vi "instrumentProperties_status.vi"(0 "reference":refnum<class "OSA.lvclass">, 5 "error in (no error)":errorcluster, 7 "poll update":bool) -> (9 "update":bool, 14 "duplicate reference":refnum<class "OSA.lvclass">, 16 "status code":u32, 17 "status":string, 18 "status struct":T1, 19 "error out":errorcluster)   [LabVIEW 2010, in "OSA.lvclass"]
doc: "Nr of samples per period depends on sensitivity mode."
uses:
  OSA.lvclass
  typeDef/status.ctl
  FTSLib.dll
  OSA20X_misc.lvlib
panel:
  out "x*2^n":u32 format="%x"
  in  "poll timeout (30s)":i32=30
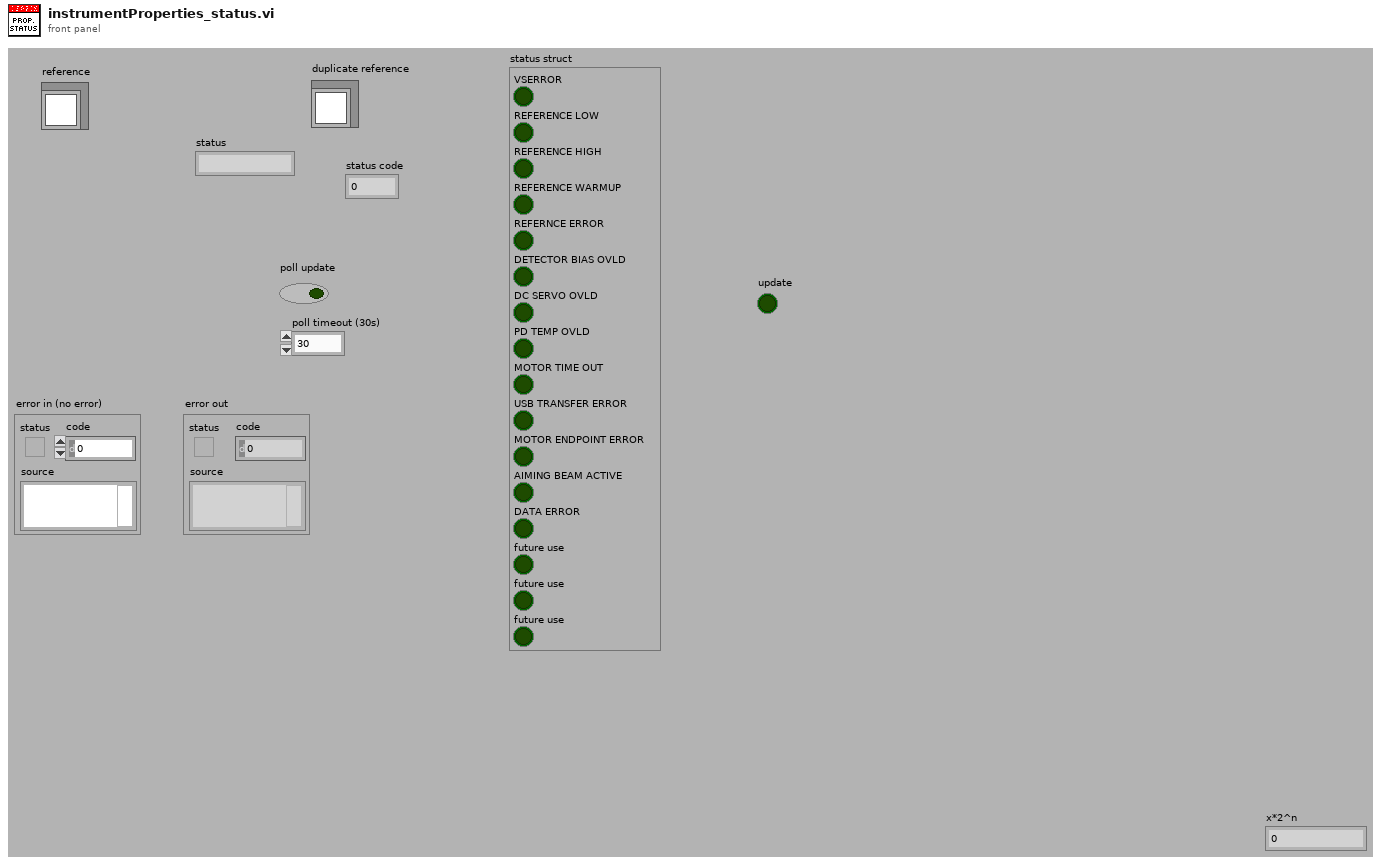
[diagram p1: front panel]
types:
  T1 = cluster{"VSERROR":bool, "REFERENCE LOW ":bool, "REFERENCE HIGH ":bool, "REFERENCE WARMUP ":bool, "REFERNCE ERROR ":bool, "DETECTOR BIAS OVLD":bool, "DC SERVO OVLD":bool, "PD TEMP OVLD":bool, "MOTOR TIME OUT":bool, "USB TRANSFER ERROR":bool, "MOTOR ENDPOINT ERROR":bool, "AIMING BEAM ACTIVE":bool, "DATA ERROR":bool, "future use":bool, "future use":bool, "future use":bool}
  T2 = typedef "OSA.lvclass/status.ctl" = cluster{"code":u32, "string":string}
  T3 = cluster{"Boolean array[0]":bool, "Boolean array[1]":bool, "Boolean array[2]":bool, "Boolean array[3]":bool, "Boolean array[4]":bool, "Boolean array[5]":bool, "Boolean array[6]":bool, "Boolean array[7]":bool, "Boolean array[8]":bool, "Boolean array[9]":bool, "Boolean array[10]":bool, "Boolean array[11]":bool, "Boolean array[12]":bool, "Boolean array[13]":bool, "Boolean array[14]":bool, "Boolean array[15]":bool}
  T4 = typedef "OSA.lvclass/ObjectAttributes.ctl" = cluster{"Stop":bool, "dataType":T5, "spectrometerIdx":u16, "buffer size interferogram":i32, "interferogram":cluster{"new":bool, "plot_x_ min":sgl, "plot_x_max":sgl, "plot_y_min":sgl, "plot_y_max":sgl, "Graph Intrfrgrm":T6, "timeStamp":u32, "signal (%)":dbl, "traces":cluster{"idx":u32, "broadBand":bool, "monoChromatic":bool, "peakToPeakSignal":dbl, "peakToPeakPos":dbl}[], "traces idx last":i32}, "spectrum":cluster{"new":bool, "plot_x_min":sgl, "plot_x_max":sgl, "plot_unit_x":T7, "plot_unit_y":T8, "plot_y_min":sgl, "plot_y_max":sgl, "Graph Spectrum":T6, "timeStamp":u32, "X_VAL_OPTIONS":enum16{"MIN_MAX", "ARRAY"}, "traces":cluster{"idx":u32}[], "traces idx last":i32}, "Thorlabs_OSA_64.lvclass:queue_action.ctlqueue ref":refnum<queue>, "action":T9, "plot zoom step":dbl, "buffer semaphore":T10, "acq stopped":bool, "dataType active":T5, "temperature (degr C)":sgl, "pressure (hPa)":sgl, "rel humidity (%)":sgl, "settings":cluster{"resolution":u16, "sensitivity":u16, "Average":bool, "average nr":u32, "apodisation":T11, "acq delay (ms)":u32, "airMesure":T12, "wmtr on":bool, "intfgrm_smooth_width":u16, "intfgrm_smooth_nrOfPasses":u16, "intfgrm_smooth":T13, "phaseCorrection":T14, "zeroFill":u8, "spectr_smooth":T13, "spectr_smooth_width":u16, "spectr_smooth_nrOfPasses":u16, "resolution (/cm)":sgl, "REF wavelength, (nm)":dbl, "gain_idx":u16, "gainAuto":bool, "gain_relative":dbl, "PD sensitivity mode":T15, "PD senseMode implemented":bool, "SensorTemperature implemented":bool, "SensorPressure implemented":bool, "SensorHumidity implemented":bool, "attenuationAuto":bool, "attenuationOnOff":bool, "attenuationAvailable":bool, "offsetAvailable":bool, "offset":i32, "offset max":u16}, "peaks position":sgl[], "peaks width":sgl[], "peaks height":sgl[], "peaks max nr":u32, "peaks latest nr":i32, "peaks new":bool, "power":dbl, "power new":bool, "path":string, "wavelength (WNr)":dbl, "wavelength new":bool, "buffer size spectrum":i32, "status":string, "VI reference":refnum<vi>, "funcPointer":u64, "libraryPointer":u64, "singleAcquisition":bool, "coherenceLength (cm)":dbl, "coherenceLength new":bool, "spectrometer model":string, "spectrometer serial nr":string, "peaks thld left":sgl[], "peaks thld right":sgl[], "coherenceLength error (cm)":dbl, "ADC bits":u16, "peaks position centroid":sgl[], "peaks height centroid":sgl[], "OSA series":T16, "channel index spectrum":u16, "spectrometer rangeLow, (/cm)":dbl, "spectrometer rangeHigh, (/cm)":dbl, "channel index interferogram":u16}
  T5 = typedef "OSA.lvclass/acq_dataType.ctl" = enum16{"none", "interferogram", "spectrum"}
  T6 = typedef "OSA.lvclass/graph_intensity.ctl" = refnum<vi>
  T7 = typedef "OSA.lvclass/spectrum_x_unit.ctl" = enum16{"wavenr/cm", "THz", "eV", "nm_air", "nm_vac"}
  T8 = typedef "OSA.lvclass/y_unit.ctl" = enum16{"ADC counts", "dBm pwr absolute", "dBm pwr density", "mW pwr absolute", "mW pwr density"}
  T9 = typedef "OSA.lvclass/queue_action.ctl" = enum16{"none", "stop", "GUI_plotInterferogram", "GUI_plotSpectrum", "GUI_plotInterferogramRescale", "GUI_plotSpectrumRescale", "GUI_plotInterferogramReset", "GUI_plotSpectrumReset", "GUI_plotInterferogramAutoScaleY", "GUI_plotSpectrumAutoScaleY", "GUI_plotInterferogramZoomOut", "GUI_plotSpectrumZoomOut", "GUI_plotInterferogramPane", "GUI_plotSpectrumPane", "GUI_plotInterferogramZoomMouse", "GUI_plotSpectrumZoomMouse", "GUI_spectrumChannelType", "GUI_channel", "ENVIRONMENT temperature", "ENVIRONMENT pressure", "MODE_resolution set", "MODE_resolution get", "MODE_sensitivity set", "MODE_sensitivity get", "MODE_PDTemperature set", "MODE_PDTemperature get", "REBOOT/RESET firmware", "ACQASYNC_acquireSingleSpectrum", "ACQASYNC_continuous start", "ACQASYNC_continuous stop\n", "ACQASYNC_get last interferogram", "ACQASYNC_get last spectrum", "ACQASYNC_get last waveNr", "ACQOPT_interferogram smoothing set", "ACQOPT_interferogram smoothing get", "ACQOPT_spectrum smoothing set", "ACQOPT_spectrum smoothing get", "ACQOPT_apodisation type set", "ACQOPT_apodisation type get", "ACQOPT_phase correction type set", "ACQOPT_phase correction type get", "ACQOPT_acqIntervall_set", "ACQOPT_acqIntervall_get", "ACQOPT_average spectrum set", "ACQOPT_average spectrum get", "ACQOPT_rolling average set", "ACQOPT_rolling average get", "ACQOPT_zero fill factor set", "ACQOPT_zero fill factor get", "ACQOPT_cycle counting set", "ACQOPT_cycle counting get", "ACQOPT_air measure option set", "ACQOPT_air measure option get", "ACQOPT_gainLevel auto get", "ACQOPT_gainLevel auto set", "ACQOPT_gainLevel get", "ACQOPT_gainLevel set", "ACQOPT_getAll", "INSTRUMENT_PROPERTY_range_WaveNr_min", "INSTRUMENT_PROPERTY_range_WaveNr_max", "INSTRUMENT_PROPERTY_reference_wavelength_cm^-1", "INSTRUMENT_PROPERTY_samplesPerRefPeriod", "INSTRUMENT_PROPERTY_resolution_waveNrPercm", "INSTRUMENT_PROPERTY_availableGainLevels", "INSTRUMENT_PROPERTY_status", "CONVERT", "ANALYSE_POWER", "ANALYSE_PEAKS", "ANALYSE_WAVELENGTH", "ANALYSE_SPECTRUM", "ANALYSE_INTERFEROGRAM", "ANALYSE_COHERENCE_LENGTH", "MATH", "MATH_power", "MATH_peaks", "FILE", "miscellaneous"}
  T10 = typedef "Semaphore RefNum" = refnum<k1>
  T11 = typedef "OSA.lvclass/apodisation.ctl" = enum16{"NONE", "NORTON_BEER_WEAK", "NORTON_BEER_MEDIUM", "NORTON_BEER_STRONG", "TRIANGULAR", "COSINE", "HANN", "HAMMING", "BLACKMANHARRIS3", "BLACKMANHARRIS4", "GAUSSIAN"}
  T12 = typedef "OSA.lvclass/airMeasure.ctl" = enum16{"TEMPERATURE", "PRESSURE"}
  T13 = typedef "OSA20X_misc.lvlib/interferogram_smoothing.ctl" = enum16{"NONE", "BINOMIAL", "SAVITSKY_GOLAY", "FOURIER", "MOVING_AVERAGE", "GAUSSIAN"}
  T14 = typedef "OSA.lvclass/phaseCorrection.ctl" = enum16{"NONE", "MERTZ", "FORMAN", "MERTZ_FILE", "FORMAN_FILE", "FUTURE COMP."}
  T15 = typedef "OSA20X_misc.lvlib/PDTemperatureMode.ctl" = enum16{"cool: better sensitivity/noise floor", "warm: extended wl range"}
  T16 = typedef "OSA.lvclass/OSA_series.ctl" = enum16{"OSA200", "OSA300", "UNKNOWN"}
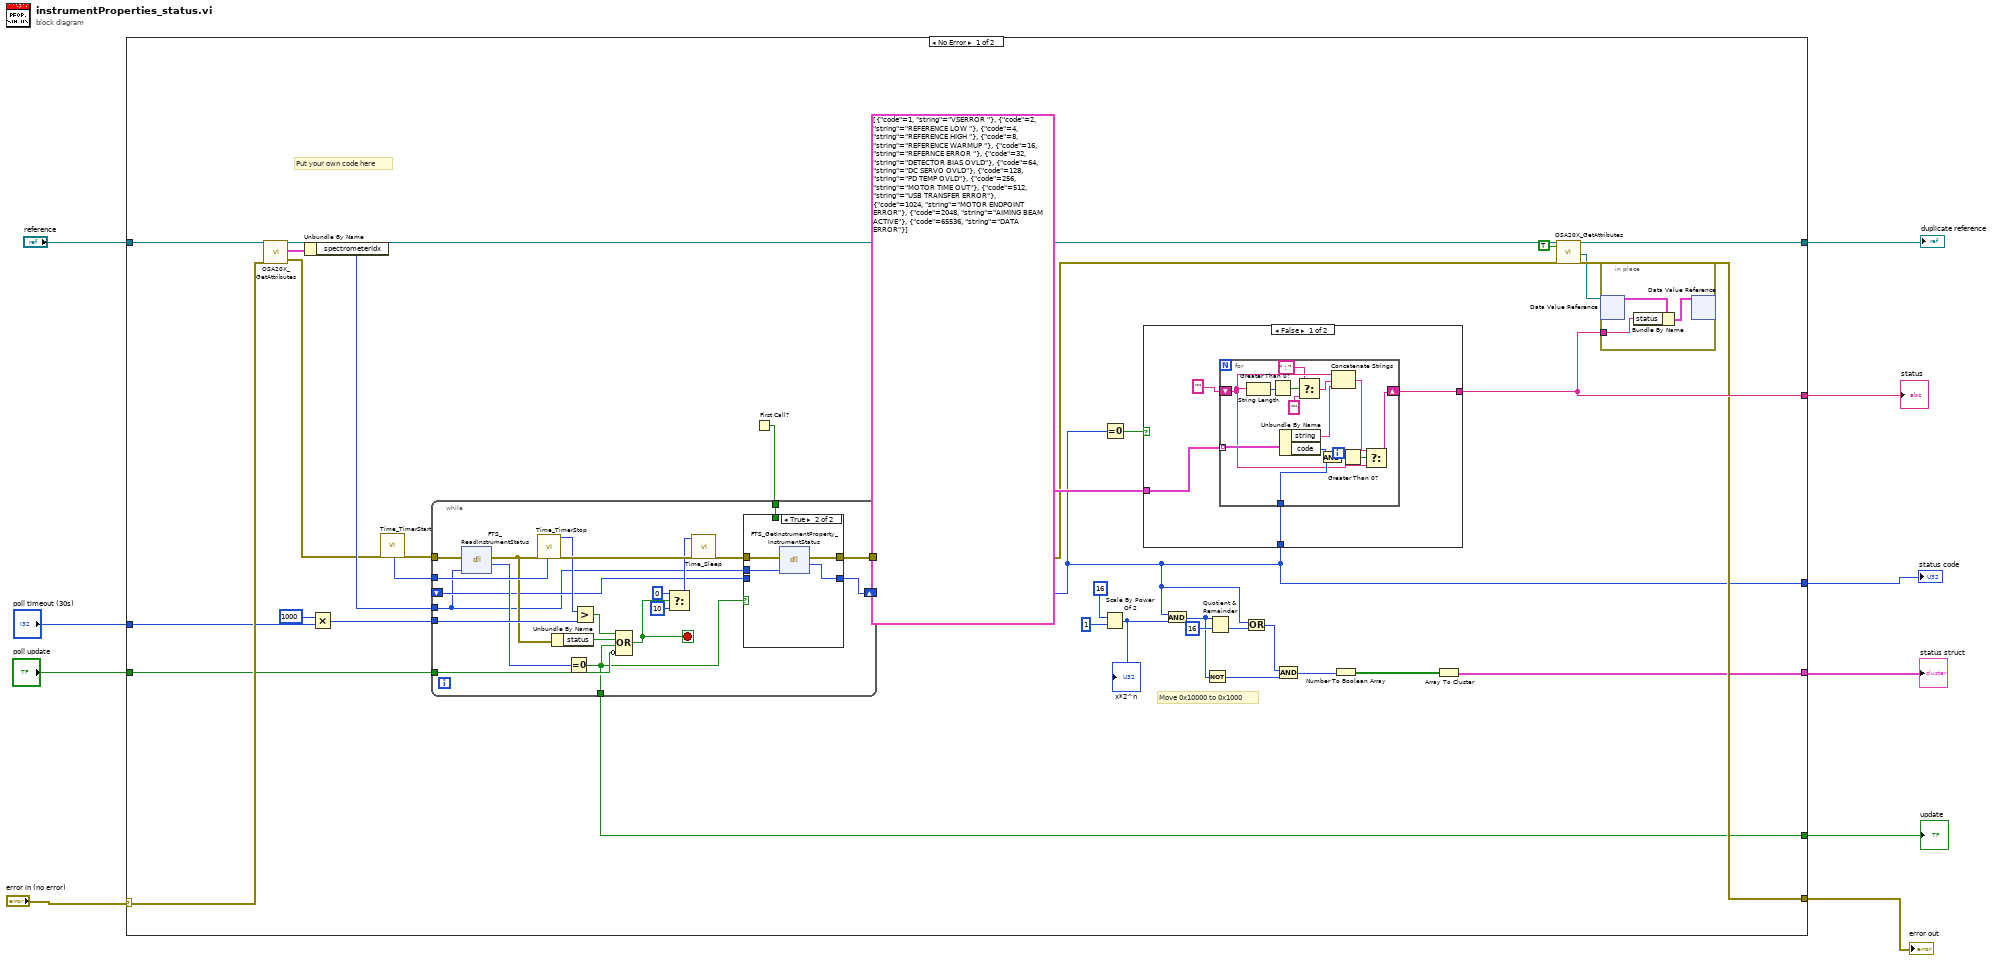
[diagram p0: block diagram]
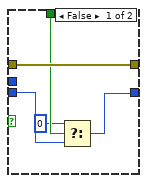
[diagram p2: hidden frame]
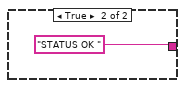
[diagram p3: hidden frame]
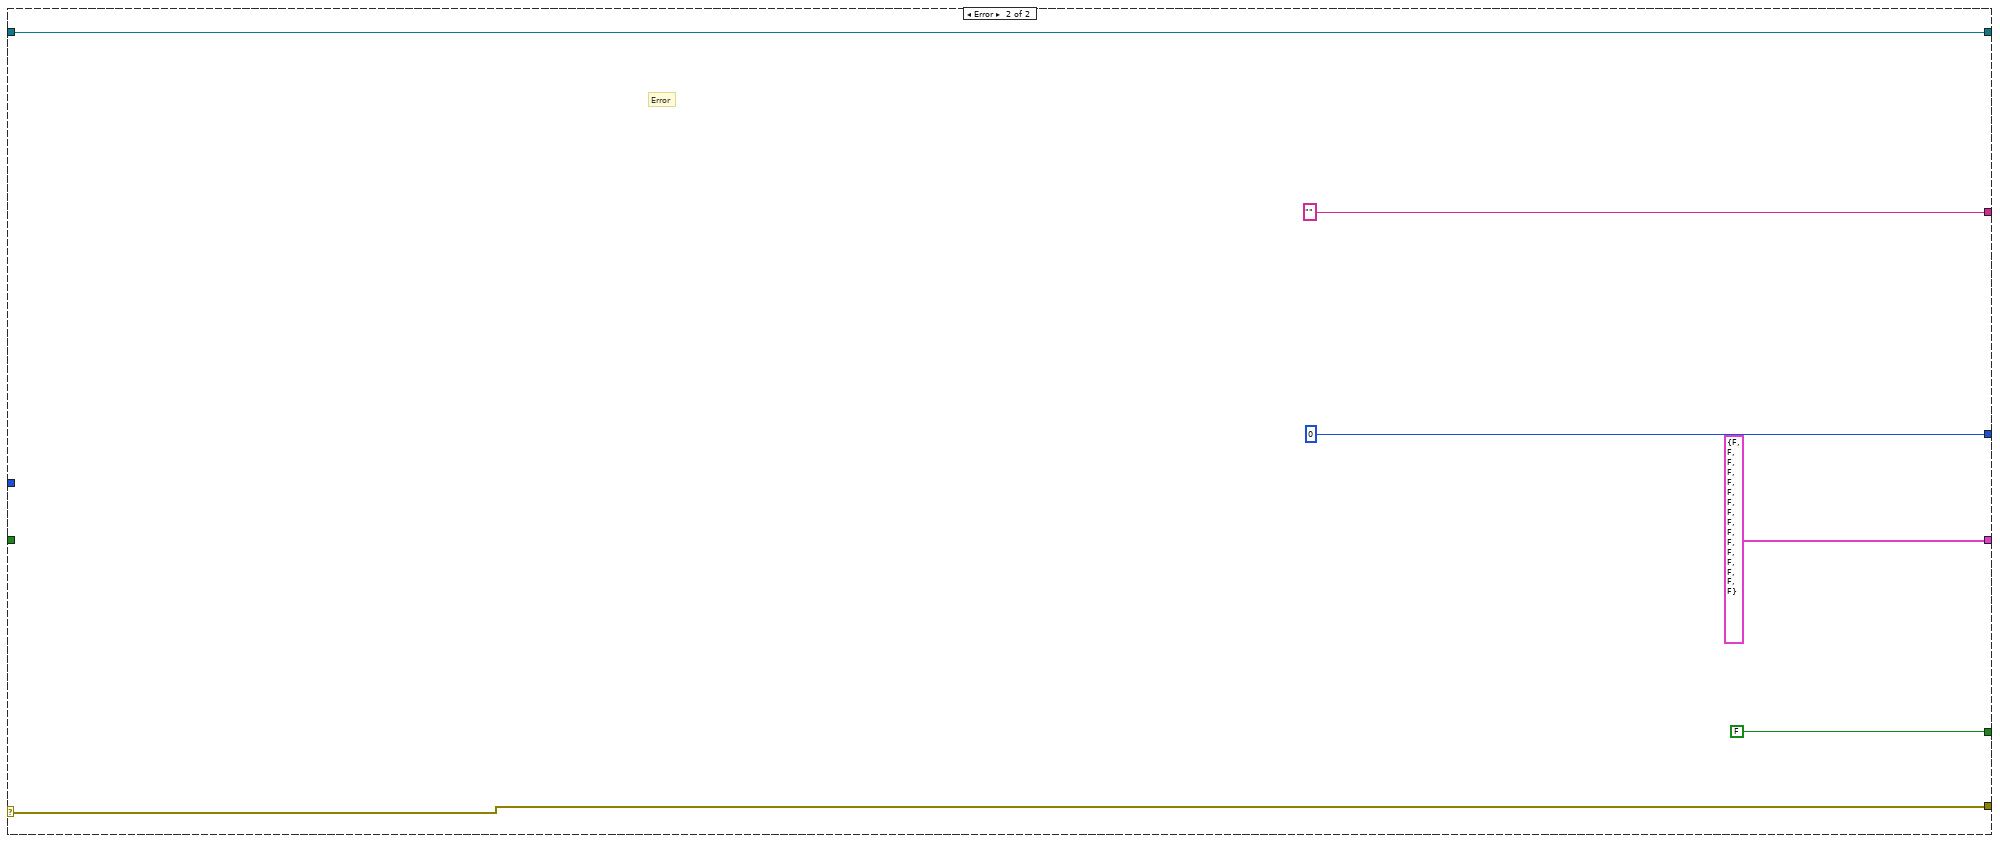
[diagram p4: hidden frame]
diagram:
  n1 = case shown="No Error" "error in (no error)" {
    selector: "error in (no error)" -> [w42 w101]
    tunnel: "reference" -> [w43 w102]
    tunnel: [w40 w101] -> w8
    tunnel: [w44 w102] -> w7
    tunnel: [w11 u32 0 ("return type")] -> w6
    tunnel: [w41 "" ("string")] -> w5
    tunnel: [w39 T3 {"Boolean array[0]"=FALSE, "Boolean array[1]"=FALSE, "Boolean array[2]"=FALSE, "Boolean array[3]"=FALSE, "Boolean array[4]"=FALSE, "Boolean array[5]"=FALSE, "Boolean array[6]"=FALSE, "Boolean array[7]"=FALSE, "Boolean array[8]"=FALSE, "Boolean array[9]"=FALSE, "Boolean array[10]"=FALSE, "Boolean array[11]"=FALSE, "Boolean array[12]"=FALSE, "Boolean array[13]"=FALSE, "Boolean array[14]"=FALSE, "Boolean array[15]"=FALSE} ("Boolean array")] -> w4
    tunnel: "poll timeout (30s)" -> [w38 _]
    tunnel: "poll update" -> [w37 _]
    tunnel: [w36 FALSE] -> w1
    frame No Error {
      # "Move 0x10000 to 0x1000"
      # "Put your own code here"
      n2 = call "OSA20X_GetAttributes.vi"("reference in"=w43, "error in (no error)"=w42) -> ("reference out"=w35:refnum<class "OSA.lvclass">, "Data"=w32:T4, "error out"=w27:errorcluster)  [unwired: 14 in, 1 out]
      n3 = Unbundle By Name(w32) -> ("spectrometerIdx"=w28:u16)
      n4 = Multiply(x=1000, y=w38) -> (x*y=w23:i32)
      n5 = call "Time_TimerStart.vi"("error in (no error)"=w27) -> ("Start Value (ms timer)"=w25:u32, "error out"=w26:errorcluster)  [unwired: 17 in]
      n6 = First Call?() -> (First Call?: T/F=w21:bool)
      n7 = while {
        tunnel: w26 -> [w65]
        tunnel: w28 -> [w46]
        tunnel: w25 -> [w63]
        tunnel: w23 -> [w60]
        tunnel: w37 -> [w53]
        tunnel: [w48] -> w36
        shift-right: [w49] -> w11
        shift-left: _ -> [w47]
        tunnel: [w50] -> w22
        tunnel: w21 -> [w45]
        stop <- w58 stop-if-true
        n8 = dll-call lib="FTSLib.dll" fn="FTS_ReadInstrumentStatus"(error in=w65, "spectrIdx"=w46) -> (error out=w54:errorcluster, "return type"=w52:i32)  [unwired: 3 in, 1 out]
        n9 = call "Time_TimerStop.vi"("error in (no error)"=w54, "Start Value (millisecond timer)"=w63) -> ("Time (millisecond timer)"=w61:i32, "error out"=w62:errorcluster)  [unwired: 16 in]
        n10 = Unbundle By Name(w54) -> ("status"=w64:bool)
        n11 = Equal To 0?(x=w52) -> (x = 0?=w48:bool)
        n12 = Greater?(x=w61, y=w60) -> (0:w59:bool)
        n13 = Compound Arithmetic op=OR(w59, w64, w48, invert w53) -> (w58:bool)
        n14 = Select(t=0, s=w58, f=10 ("Delay (msec)")) -> (s? t:f=w55:i32)
        n15 = call "Time_Sleep.vi"("Delay (msec)"=w55, "error in (no error)"=w62) -> ("error out"=w51:errorcluster)  [unwired: 17 in]
        n16 = case shown="True" w48 {
          tunnel: w51 -> [w70 w74]
          tunnel: [w70 w73] -> w50
          tunnel: [w66 w72] -> w49
          tunnel: w47 -> [w68 _]
          tunnel: w46 -> [_ w71]
          tunnel: w45 -> [w69 _]
          frame False {
            n17 = Select(t=u32 0, s=w69, f=w68) -> (s? t:f=w66:u32)
          }
          frame True {
            n18 = dll-call lib="FTSLib.dll" fn="FTS_GetInstrumentProperty_InstrumentStatus"(error in=w74, "spectrIdx"=w71) -> (error out=w73:errorcluster, "return type"=w72:u32)  [unwired: 3 in, 1 out]
          }
        }
      }
      n19 = Scale By Power Of 2(n=i16 16, x=u32 1 ("unsigned 32bit integer")) -> (x*2^n=w18:u32)
      "x*2^n" <- w18
      n20 = Equal To 0?(x=w11) -> (x = 0?=w30:bool)
      n21 = case shown="False" w30 {
        tunnel: T2[] [{"code"=1, "string"="VSERROR "}, {"code"=2, "string"="REFERENCE LOW "}, {"code"=4, "string"="REFERENCE HIGH "}, {"code"=8, "string"="REFERENCE WARMUP "}, {"code"=16, "string"="REFERNCE ERROR "}, {"code"=32, "string"="DETECTOR BIAS OVLD"}, {"code"=64, "string"="DC SERVO OVLD"}, {"code"=128, "string"="PD TEMP OVLD"}, {"code"=256, "string"="MOTOR TIME OUT"}, {"code"=512, "string"="USB TRANSFER ERROR"}, {"code"=1024, "string"="MOTOR ENDPOINT ERROR"}, {"code"=2048, "string"="AIMING BEAM ACTIVE"}, {"code"=65536, "string"="DATA ERROR"}] ("stat") -> [w78 _]
        tunnel: w11 -> [w77 _]
        tunnel: [w75 "STATUS OK " ("string")] -> w41
        frame False {
          n22 = for {
            tunnel: w78 -> [w92] mode=indexing
            tunnel: w77 -> [w90]
            shift-right: [w89] -> w75
            shift-left: "" ("string") -> [w85]
            n23 = String Length(string=w85) -> (length=w84:i32)
            n24 = Greater Than 0?(x=w84) -> (x > 0?=w83:bool)
            n25 = Unbundle By Name(w92) -> ("string"=w79:string, "code"=w91:u32)
            n26 = Select(t=" : " ("string"), s=w83, f="" ("string")) -> (s? t:f=w81:string)
            n27 = And(x=w91, y=w90) -> (x .and. y?=w88:u32)
            n28 = Concatenate Strings(w85, w81, w79) -> (w86:string)
            n29 = Greater Than 0?(x=w88) -> (x > 0?=w87:bool)
            n30 = Select(t=w86, s=w87, f=w85) -> (s? t:f=w89:string)
          }
        }
        frame True {
        }
      }
      n31 = And(x=w11, y=w18) -> (x .and. y?=w15:u32)
      n32 = Not(x=w15) -> (.not. x?=w14:u32)
      n33 = Quotient & Remainder(x=w15, y=u32 16) -> (floor(x/y)=w16:u32)  [unwired: 1 out]
      n34 = Or(x=w11, y=w16) -> (x .or. y?=w13:u32)
      n35 = And(x=w13, y=w14) -> (x .and. y?=w12:u32)
      n36 = Number To Boolean Array(number=w12) -> (Boolean array=w29:bool[])
      n37 = Array To Cluster(array=w29) -> (cluster=w39:T3)
      n38 = call "OSA20X_GetAttributes.vi"("reference in"=w35, "OnlyGetDvrReference(False)"=TRUE, "error in (no error)"=w22) -> ("reference out"=w44:refnum<class "OSA.lvclass">, "DataRef"=w31:refnum<data-value>, "error out"=w40:errorcluster)  [unwired: 13 in, 1 out]
      n39 = in-place {
        in-place-border: w41 -> [w95]
        n40 = in-place-dvr #1(w31) -> (w96:T4)  [unwired: 1 out]
        n41 = Bundle By Name(cluster=w96, "status"=w95) -> (w94:T4)
        n42 = in-place-dvr #1(w94) -> ()  [unwired: 2 out]
      }
    }
    frame Error {
      # "Error"
    }
  }
  "error out" <- w8
  "duplicate reference" <- w7
  "status code" <- w6
  "status" <- w5
  "status struct" <- w4
  "update" <- w1
